vi "Perform_Pulse_Integral_Analysis.vi"(6 "Tail Integral":dbl[](array[numeric]), 9 "Total Integral":dbl[](array[numeric]), 11 "IntensityGraph in":refnum<vi>) -> (1 "Scatter plot":cluster{"Array":dbl[], "Array":dbl[]}, 2 "Histogram":u32[](array[numeric]), 3 "Intensity graph":u32[][](array[numeric]))   [LabVIEW 2015]
uses:
  ESA_Data_Analysis_Global_VIs.vi
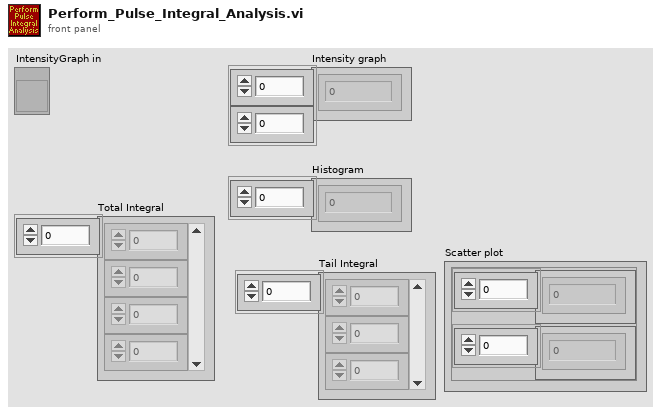
[diagram p1: front panel]
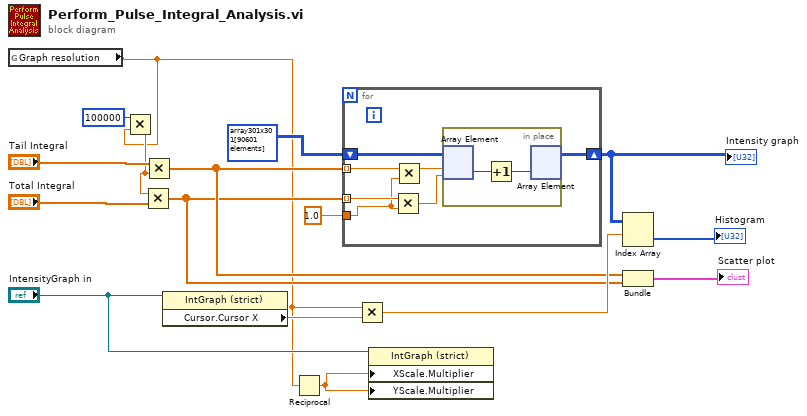
[diagram p0: block diagram]
diagram:
  n1 = global read "ESA_Data_Analysis_Global_VIs.vi" "Graph resolution"() -> (w1:dbl)
  n2 = Multiply(x=100000, y=w1) -> (x*y=w2:dbl)
  n3 = Multiply(x=w2, y="Total Integral") -> (x*y=w4:dbl[])
  n4 = Multiply(x="Tail Integral", y=w2) -> (x*y=w5:dbl[])
  n5 = property on="Property Node" class="IntGraph (strict)"(reference="IntensityGraph in") -> ("Cursor.Cursor X"=w15:dbl)  [unwired: 1 in, 2 out]
  n6 = Reciprocal(x=w1) -> (1/x=w7:dbl)
  n7 = for {
    shift-right: [w22] -> w13
    shift-left: u32[][] array301x301[90601 elements] -> [w23]
    tunnel: w5 -> [w21] mode=indexing
    tunnel: w4 -> [w20] mode=indexing
    tunnel: 1.0 ("Graph resolution") -> [w17]
    n8 = Multiply(x=w20, y=w17) -> (x*y=w18:dbl)
    n9 = Multiply(x=w21, y=w17) -> (x*y=w19:dbl)
    n10 = in-place {
      n11 = in-place-array #1(w23, w19, w18) -> (w25:u32)
      n12 = Increment(x=w25) -> (x+1=w24:u32)
      n13 = in-place-array #1(w24) -> (w22:u32[][])  [unwired: 2 out]
    }
  }
  "Intensity graph" <- w13
  n14 = Multiply(x=w1, y=w15) -> (x*y=w16:dbl)
  n15 = property on="Property Node" class="IntGraph (strict)"(reference="IntensityGraph in", "XScale.Multiplier"=w7, "YScale.Multiplier"=w7) -> ()  [unwired: 1 in, 2 out]
  n16 = Index Array(array=w13, index (row)=w16) -> (element=→"Histogram":u32[])  [unwired: 1 in]
  n17 = Bundle(w5, w4) -> (→"Scatter plot":cluster{dbl[], dbl[]})  [unwired: 1 in]
